vi "Demo 1 - Image Gallery - Check Image Type.vi"(8 "error in":errorcluster, 11 "Image Path In":path) -> (0 "error out":errorcluster, 2 "Image Type Out":T1, 3 "Image Path Out":path)   [LabVIEW 2011]
uses:
  Controls/ImageType.ctl
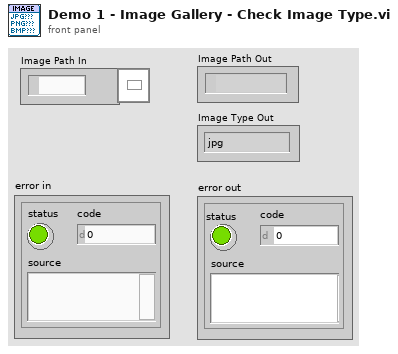
[diagram p1: front panel]
types:
  T1 = typedef "ImageType.ctl" = enum16{"jpg", "png", "bmp"}
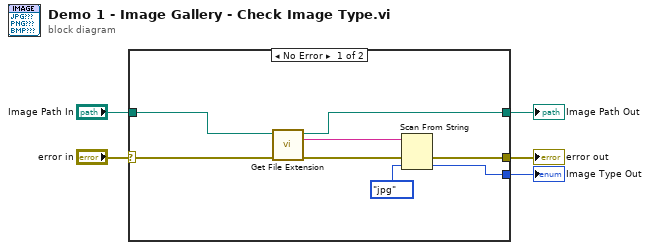
[diagram p0: block diagram]
diagram:
  n1 = case shown="No Error" "error in" {
    selector: "error in" -> [w10 w14]
    tunnel: "Image Path In" -> [w8 _]
    tunnel: [w12 w14] -> w4
    tunnel: [w11 _] -> w3
    tunnel: [w7 _] -> w1
    frame No Error {
      n2 = call <vilib>:"Get File Extension.vi"("error in (no error)"=w10, "file"=w8) -> ("error out"=w9:errorcluster, "lowercase file extension"=w6:string, "dup file"=w7:path)  [unwired: 6 in, 1 out]
      n3 = Scan From String(input string=w6, error in=w9, default 1=ImageType."jpg") -> (error out=w12:errorcluster, output 1=w11:T1)  [unwired: 2 in, 2 out]
    }
    frame Error {
    }
  }
  "error out" <- w4
  "Image Type Out" <- w3
  "Image Path Out" <- w1
